vi "Read Channel Controllers.vi"(8 "error in (no error)":errorcluster, 11 "Interface in":refnum<class "Interface.lvclass">) -> (0 "error out":errorcluster, 3 "Interface out":refnum<class "Interface.lvclass">)   [LabVIEW 2018, in "Interface.lvclass"]
uses:
  Interface.lvclass
  Interface.lvclass/Interface.ctl
panel:
  out "Channel Controllers":T1
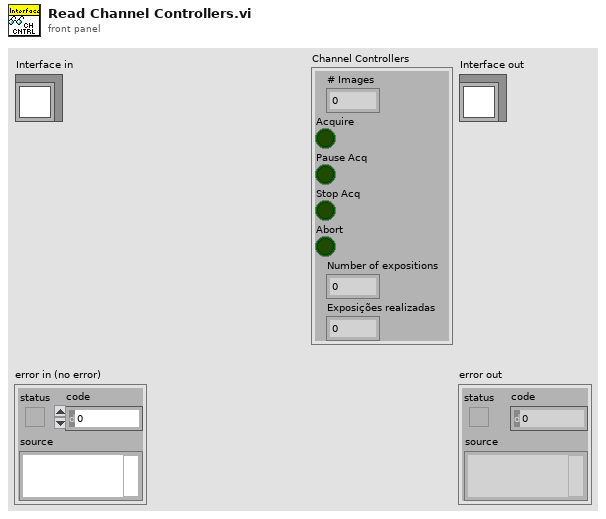
[diagram p1: front panel]
types:
  T1 = cluster{"# Images":u32, "Acquire":bool, "Pause Acq":bool, "Stop Acq":bool, "Abort":bool, "Number of expositions":dbl, "Exposições realizadas":dbl}
  T2 = cluster{"Cubes":u32, "Acquire":bool, "Pause Acq":bool, "Stop Acq":bool, "Abort":bool, "Number of expositions":dbl, "Exposições realizadas":dbl}
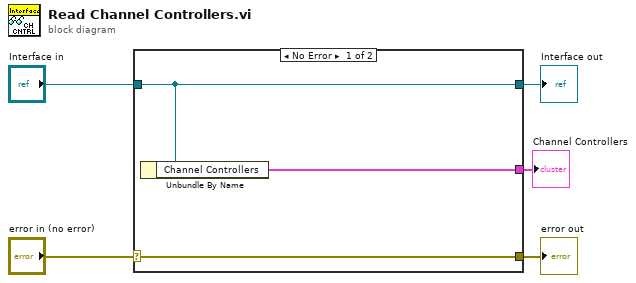
[diagram p0: block diagram]
diagram:
  n1 = case shown="No Error" "error in (no error)" {
    selector: "error in (no error)" -> [w8 w9]
    tunnel: [w8 w9] -> w4
    tunnel: [w7 w10] -> w2
    tunnel: "Interface in" -> [w7 w10]
    tunnel: [w6 _] -> w1
    frame No Error {
      n2 = Unbundle By Name(w7) -> ("Channel Controllers"=w6:T2)
    }
    frame Error {
    }
  }
  "error out" <- w4
  "Interface out" <- w2
  "Channel Controllers" <- w1
